vi "CLD 9 Step Sequencer Express Timer Front Panel.vi"() -> ()   [LabVIEW 2014]
doc: "CLD-Übung 9"
panel:
  out "Dauer des aktuellen Schritts":dbl
  out "Verstrichene Zeit (s)":string
  out "Schritt 3":bool
  out "Schritt 2":bool
  out "Schritt 1":bool
  out "Zeit ist verstrichen":bool
  in  "Autom. zurücksetzen":bool=TRUE
  in  "Zurücksetzen-Schaltfläche":bool
  in  "VI anhalten":bool
  out "Fehler (Ausgang)":errorcluster
  in  "Fehler (Eingang, kein Fehler)":errorcluster
  in  "Zielzeit (s)":dbl
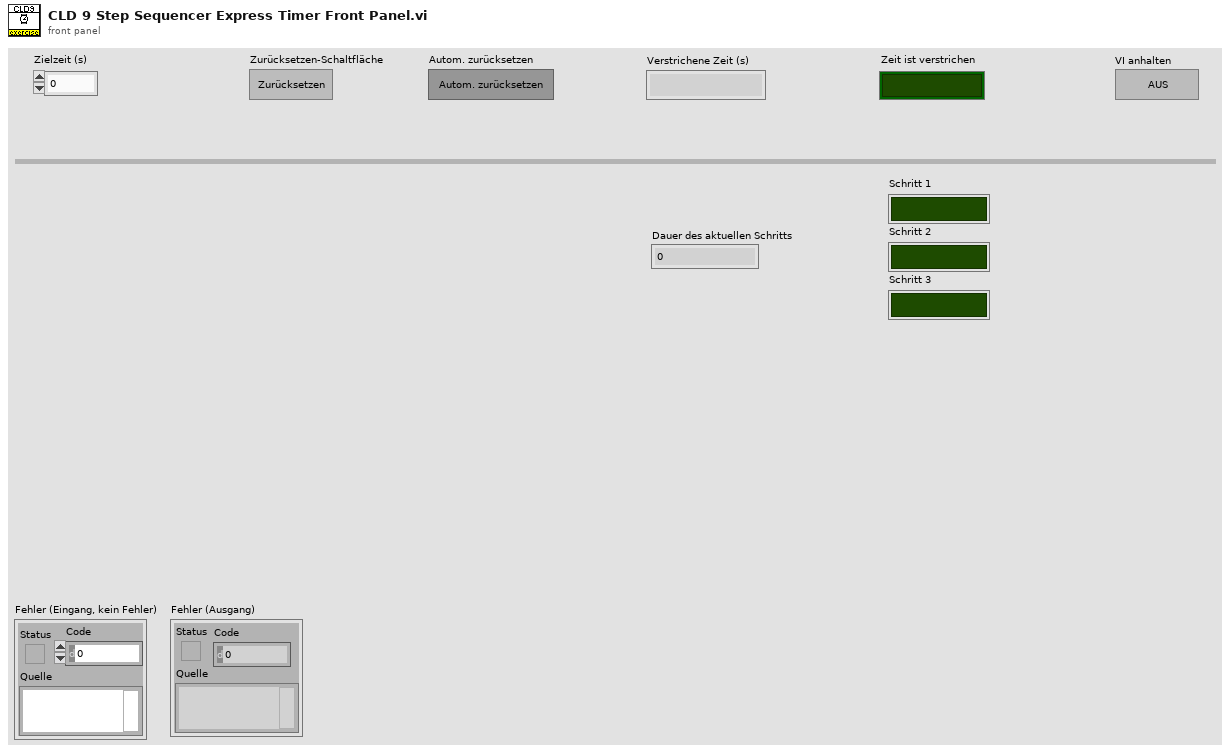
[diagram p1: front panel]
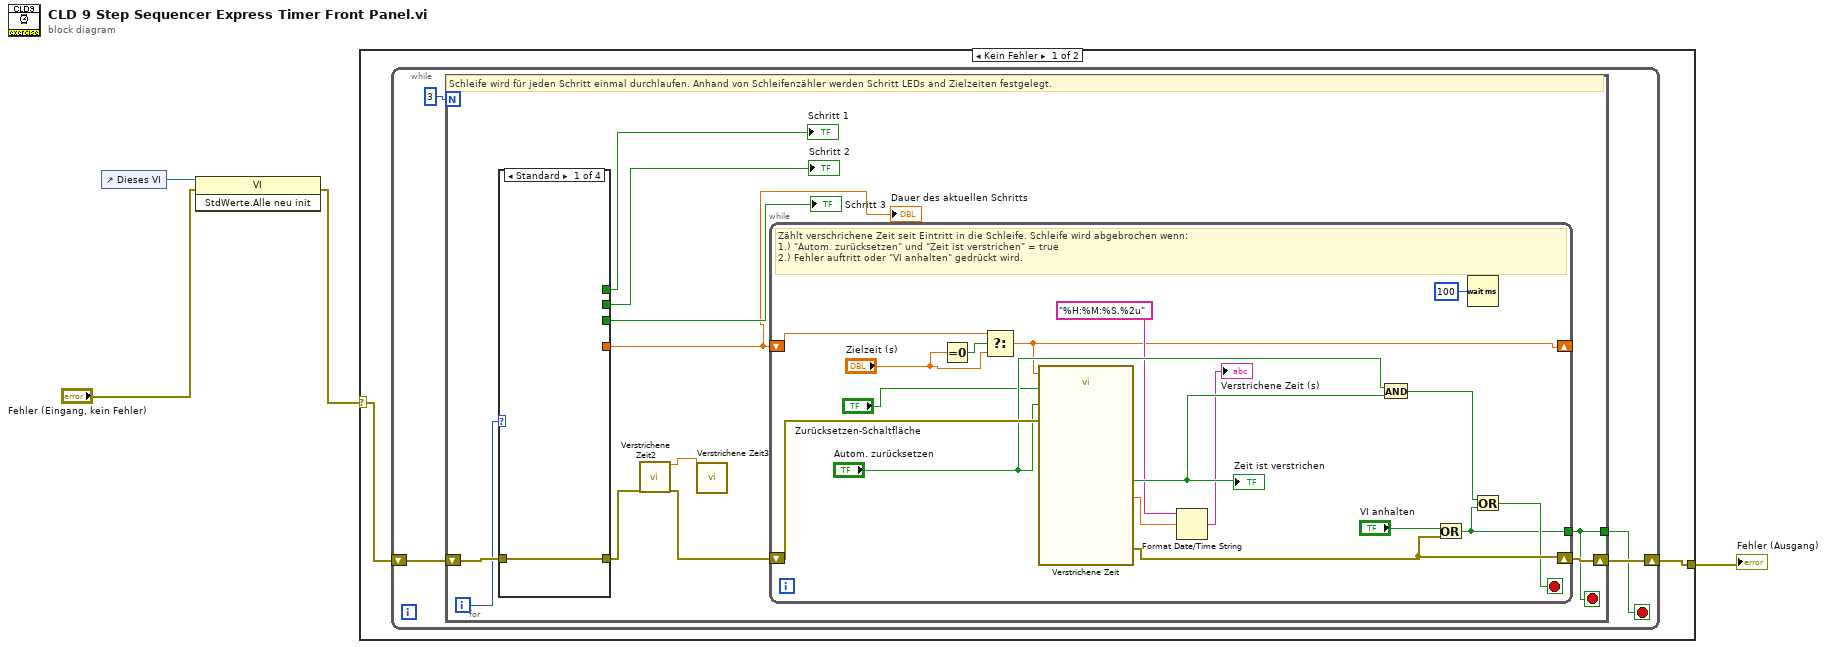
[diagram p0: block diagram]
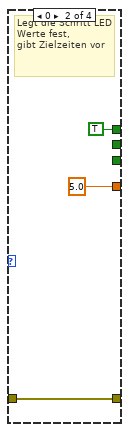
[diagram p2: hidden frame]
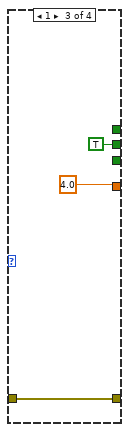
[diagram p3: hidden frame]
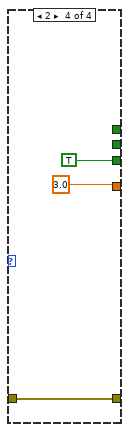
[diagram p4: hidden frame]
diagram:
  n1 = control-ref of="Dieses VI"() -> (w3:refnum<vi>)
  n2 = invoke class="VI" method="StdWerte.Alle neu init"(reference=w3, error in="Fehler (Eingang, kein Fehler)") -> (error out=w1:errorcluster)  [unwired: 1 in, 2 out]
  n3 = case shown="Kein Fehler" w1 {
    selector: w1 -> [w5 w49]
    tunnel: [w6 w49] -> w4
    frame No Error {
      n4 = while {
        shift-right: [w10] -> w6
        shift-left: w5 -> [w9]
        stop <- w7 stop-if-true
        n5 = for {
          N: 3 -> [_]
          shift-right: [w21] -> w10
          shift-left: w9 -> [w20]
          tunnel: [w15] -> w7
          i -> [w11]
          stop <- w15 stop-if-true
          # "Schleife wird für jeden Schritt einmal durchlaufen. Anhand von Schleifenzähler werden Schritt LEDs and Zielzeiten festgelegt."
          n6 = case shown="Standard" w11 {
            tunnel: [_ 5.0 4.0 3.0] -> w16
            tunnel: w20 -> [w22 w24 w27 w30]
            tunnel: [w22 w24 w27 w30] -> w14
            tunnel: [_ TRUE ("Schritt 1") _ _] -> w19
            tunnel: [_ _ TRUE ("Schritt 1") _] -> w18
            tunnel: [_ _ _ TRUE ("Schritt 1")] -> w17
            frame Default {
            }
            frame 0 {
              # "Legt die Schritt LED Werte fest,\ngibt Zielzeiten vor"
            }
            frame 1 {
            }
            frame 2 {
            }
          }
          "Schritt 1" <- w19
          "Schritt 2" <- w18
          "Schritt 3" <- w17
          "Dauer des aktuellen Schritts" <- w16
          n7 = call "Verstrichene Zeit2"("error in (no error)"=w14) -> ("Present (s)"=w12:dbl, "error out"=w13:errorcluster)  [unwired: 11 in, 6 out]
          n8 = call "Verstrichene Zeit3"("Set Start Time (s)"=w12) -> ()  [unwired: 11 in, 8 out]
          n9 = while {
            shift-right: [w46] -> w21
            shift-left: w13 -> [w48]
            tunnel: [w38] -> w15
            shift-right: [w33] -> _
            shift-left: w16 -> [w44]
            stop <- w40 stop-if-true
            # "Zählt verschrichene Zeit seit Eintritt in die Schleife. Schleife wird abgebrochen wenn:\n1.) \"Autom. zurücksetzen\" und \"Zeit ist verstrichen\" = true\n2.) Fehler auftritt oder \"VI anhalten\" gedrückt wird."
            n10 = Equal To 0?(x="Zielzeit (s)") -> (x = 0?=w45:bool)
            n11 = Select(t=w44, s=w45, f="Zielzeit (s)") -> (s? t:f=w33:dbl)
            n12 = call "Verstrichene Zeit"("Time Target (s)"=w33, "Reset"="Zurücksetzen-Schaltfläche", "Auto Reset"="Autom. zurücksetzen", "error in (no error)"=w48) -> ("Elapsed Time (s)"=w37:dbl, "Time has Elapsed"=w41:bool, "error out"=w46:errorcluster)  [unwired: 8 in, 5 out]
            "Zeit ist verstrichen" <- w41
            n13 = Format Date/Time String(time format string (%c)="%H:%M:%S.%2u" ("Zeitformatierungs-String (%c)"), seconds (now)=w37) -> (date/time string=→"Verstrichene Zeit (s)":string)  [unwired: 1 in]
            n14 = And(x="Autom. zurücksetzen", y=w41) -> (x .and. y?=w39:bool)
            n15 = Or(x="VI anhalten", y=w46) -> (x .or. y?=w38:bool)
            n16 = Wait (ms)(milliseconds to wait=u32 100 ("Zu wartende ms")) -> ()  [unwired: 1 out]
            n17 = Or(x=w39, y=w38) -> (x .or. y?=w40:bool)
          }
        }
      }
    }
    frame Error {
    }
  }
  "Fehler (Ausgang)" <- w4
